vi "OAT State Machine Generate Events for Booleans.vi"(1 "Initialize":bool, 2 "Booleans":bool[](array[boolean]), 4 "Event":T1(array[ring])) -> (7 "Event Found?":bool[](array[boolean]))   [LabVIEW 2017]
doc: "Detects events for the boolean objects. The event of boolean range from true, false,true to false, false to true and boolean crossing. When the event detected, the coresponding output boolean is TRUE."
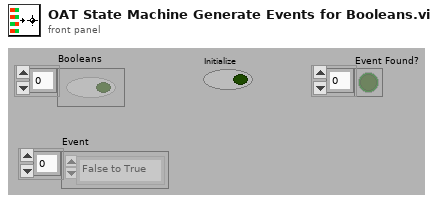
[diagram p1: front panel]
types:
  T1 = enum16{"False to True", "True to False", "Either Crossing", "True", "False"}[]
  T2 = enum16{"False to True", "True to False", "Either Crossing", "True", "False"}
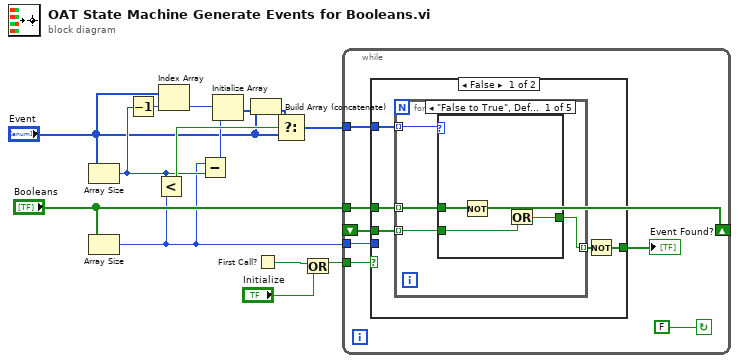
[diagram p0: block diagram]
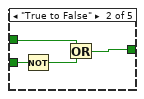
[diagram p2: hidden frame]
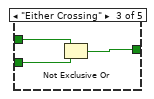
[diagram p3: hidden frame]
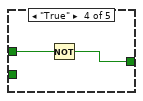
[diagram p4: hidden frame]
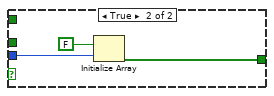
[diagram p6: hidden frame]
diagram:
  n1 = Array Size(array="Event") -> (size(s)=w11:i32)
  n2 = Array Size(array="Booleans") -> (size(s)=w4:i32)
  n3 = Decrement(x=w11) -> (x-1=w12:i32)
  n4 = Less?(x=w11, y=w4) -> (x < y?=w13:bool)
  n5 = Index Array(array="Event", index=w12) -> (element=w14:T2)
  n6 = Subtract(x=w4, y=w11) -> (x-y=w10:i32)
  n7 = Initialize Array(w14, w10) -> (w8:T1)
  n8 = Build Array (concatenate)("Event", w8) -> (w9:T1)
  n9 = First Call?() -> (First Call?: T/F=w3:bool)
  n10 = Select(t=w9, s=w13, f="Event") -> (s? t:f=w7:T1)
  n11 = Or(x=w3, y="Initialize") -> (x .or. y?=w2:bool)
  n12 = while {
    tunnel: w4 -> [w15]
    tunnel: w2 -> [w16]
    tunnel: "Booleans" -> [w19]
    shift-left: _ -> [w20]
    shift-right: [w19] -> _
    tunnel: w7 -> [w21]
    stop <- FALSE continue-if-true
    n13 = case shown="False" w16 {
      tunnel: w21 -> [w26 _]
      tunnel: w20 -> [w25 _]
      tunnel: w19 -> [w24 _]
      tunnel: [w22 w45] -> w17
      tunnel: w15 -> [_ w47]
      frame False {
        n14 = for {
          tunnel: w26 -> [w30] mode=indexing
          tunnel: w25 -> [w28] mode=indexing
          tunnel: w24 -> [w29] mode=indexing
          tunnel: [w27] -> w23 mode=indexing
          n15 = case shown="\"False to True\", Default" w30 {
            tunnel: w29 -> [w34 w36 w41 w43 w44]
            tunnel: w28 -> [w32 w38 w40 _ _]
            tunnel: [w31 w35 w39 w42 w44] -> w27
            frame "False to True", Default {
              n16 = Not(x=w34) -> (.not. x?=w33:bool)
              n17 = Or(x=w33, y=w32) -> (x .or. y?=w31:bool)
            }
            frame "True to False" {
              n18 = Not(x=w38) -> (.not. x?=w37:bool)
              n19 = Or(x=w36, y=w37) -> (x .or. y?=w35:bool)
            }
            frame "Either Crossing" {
              n20 = Not Exclusive Or(1:w40, 2:w41) -> (0:w39:bool)
            }
            frame "True" {
              n21 = Not(x=w43) -> (.not. x?=w42:bool)
            }
            frame "False" {
            }
          }
        }
        n22 = Not(x=w23) -> (.not. x?=w22:bool[])
      }
      frame True {
        n23 = Initialize Array(FALSE, w47) -> (w45:bool[])
      }
    }
    "Event Found?" <- w17
  }
